vi "mainog_instant write.vi"() -> ()   [LabVIEW 2014]
uses:
  <vilib>/Instr/_visa.llb/VISA Configure Serial Port (Instr).vi
panel:
  out "Numeric":u32
  out "12bit DAC signal sent 2":string
  in  "Keep Data?":bool
  out "12bit DAC signal sent":string
  in  "filepath:":path
  out "Pressure Plot":i32[](graph)
  in  "Desired Pressures":dbl[](array[numeric])
  out "mbar":string[](array[string])
  out "status":bool
  out "error out":errorcluster
  in  "error in":errorcluster
  in  "stop":bool
  # "Arduino LabVIEW - Serial Read and Write"
  # "Measured Pressures"
  # "Desired pressures must be expressed in volts (0-5)"
  # "Channel 1"
  # "Channel 2"
  # "Channel 1"
  # "Channel 3"
  # "Channel 2"
  # "Channel 4"
  # "Channel 3"
  # "Channel 4"
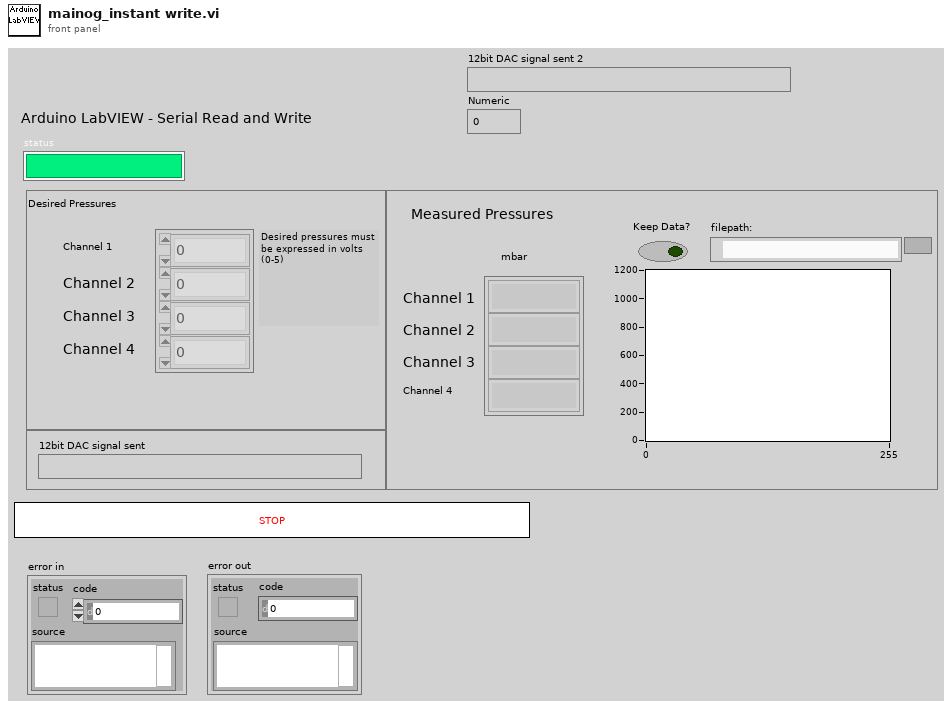
[diagram p1: front panel]
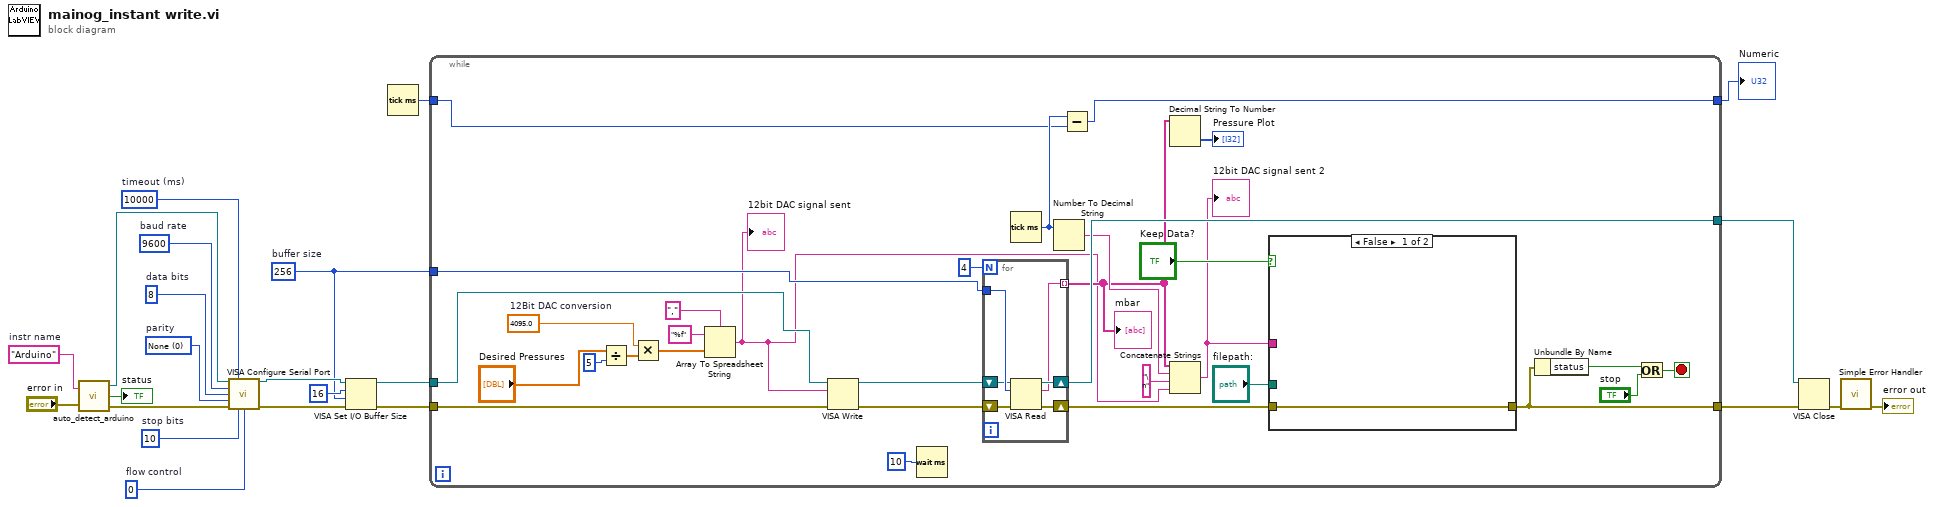
[diagram p0: block diagram]
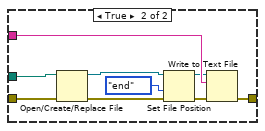
[diagram p2: hidden frame]
diagram:
  w14 = "Arduino"  # instr name
  w8 = u32 256  # buffer size
  w21 = u16 0  # flow control
  w20 = u16 10  # stop bits
  w19 = u16 0 items=["None", "Odd", "Even", "Mark", "Space"]  # parity
  w18 = u16 8  # data bits
  w17 = u32 9600  # baud rate
  w22 = u32 10000  # timeout (ms)
  n1 = call "auto_detect_arduino.vi"("instr name"=w14, "error in"="error in") -> ("VISA resource name"=w16:refnum<visa-resource-name>, "status"=→"status":bool, "error out"=w15:errorcluster)
  n2 = call-poly "VISA Configure Serial Port"("VISA resource name"=w16, "timeout (10sec)"=w22, "baud rate (9600)"=w17, "data bits (8)"=w18, "parity (0:none)"=w19, "error in (no error)"=w15, "stop bits (10: 1 bit)"=w20, "flow control (0:none)"=w21) -> ("VISA resource name out"=w12:refnum<visa-resource-name>, "error out"=w11:errorcluster)  [unwired: 6 in]
  n3 = VISA Set I/O Buffer Size(VISA resource name=w12, mask (16)=u16 16 ("I/O Receive\nBuffer mask"), size (4096)=w8, error in (no error)=w11) -> (VISA resource name out=w10:refnum<visa-resource-name>, error out=w9:errorcluster)
  n4 = Tick Count (ms)() -> (millisecond timer value=w2:u32)
  n5 = while {
    tunnel: w10 -> [w25]
    tunnel: w9 -> [w28]
    tunnel: [w51] -> w23
    tunnel: w8 -> [w52]
    tunnel: [w39] -> w3
    tunnel: w2 -> [w30]
    tunnel: [w29] -> w1
    stop <- w53 stop-if-true
    w42 = 4095.0  # 12Bit DAC conversion
    n6 = Divide(x="Desired Pressures", y=5) -> (x/y=w44:dbl[])
    n7 = Multiply(x=w42, y=w44) -> (x*y=w43:dbl[])
    n8 = Array To Spreadsheet String(delimiter (Tab)=",", array=w43, 3:"%f" ("format string")) -> (spreadsheet string=w24:string)
    "12bit DAC signal sent" <- w24
    n9 = VISA Write(VISA resource name=w25, write buffer=w24, error in (no error)=w28) -> (VISA resource name out=w26:refnum<visa-resource-name>, error out=w27:errorcluster)  [unwired: 1 out]
    n10 = Wait (ms)(milliseconds to wait=u32 10) -> ()  [unwired: 1 out]
    n11 = for {
      N: 4 -> [_]
      tunnel: w52 -> [w69]
      tunnel: [w65] -> w32 mode=indexing
      shift-right: [w68] -> w51
      shift-left: w26 -> [w67]
      shift-right: [w70] -> w40
      shift-left: w27 -> [w66]
      n12 = VISA Read(VISA resource name=w67, byte count=w69, error in (no error)=w66) -> (VISA resource name out=w68:refnum<visa-resource-name>, read buffer=w65:string, error out=w70:errorcluster)  [unwired: 1 out]
    }
    "mbar" <- w32
    n13 = Tick Count (ms)() -> (millisecond timer value=w31:u32)
    n14 = Number To Decimal String(number=w31) -> (decimal integer string=w33:string)  [unwired: 1 in]
    n15 = Subtract(x=w31, y=w30) -> (x-y=w29:u32)
    n16 = Decimal String To Number(string=w32) -> (number=→"Pressure Plot":i32[])  [unwired: 2 in, 1 out]
    n17 = Concatenate Strings(w32, w33, "\n" ("string"), w24) -> (w35:string)
    "12bit DAC signal sent 2" <- w35
    n18 = case shown="False" "Keep Data?" {
      tunnel: w35 -> [_ w64]
      tunnel: "filepath:" -> [_ w63]
      tunnel: w40 -> [w55 w62]
      tunnel: [w55 w57] -> w39
      frame False {
      }
      frame True {
        n19 = Open/Create/Replace File(file path (use dialog)=w63, error in=w62) -> (refnum out=w60:refnum<file>, error out=w61:errorcluster)  [unwired: 4 in, 1 out]
        n20 = Set File Position(refnum=w60, from (0:start)=enum16{"start", "end", "current"}."end", error in=w61) -> (refnum out=w59:refnum<file>, error out=w58:errorcluster)  [unwired: 1 in]
        n21 = Write to Text File(file (use dialog)=w59, text=w64, error in=w58) -> (error out=w57:errorcluster)  [unwired: 1 in, 2 out]
      }
    }
    n22 = Unbundle By Name(w39) -> ("status"=w38:bool)
    n23 = Or(x=w38, y="stop") -> (x .or. y?=w53:bool)
  }
  "Numeric" <- w1
  n24 = VISA Close(VISA resource name=w23, error in (no error)=w3) -> (error out=w6:errorcluster)
  n25 = call <vilib>:"Simple Error Handler.vi"("error in (no error)"=w6) -> ("error out"=→"error out":errorcluster)  [unwired: 4 in, 4 out]
